vi "CoerceToRange.vi"(10 "Range":T1, 11 "input":dbl) -> (3 "coerced":dbl)   [LabVIEW 2017]
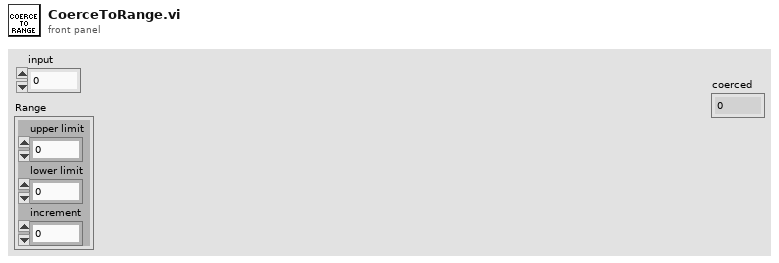
[diagram p1: front panel]
types:
  T1 = cluster{"upper limit":dbl, "lower limit":dbl, "increment":dbl}
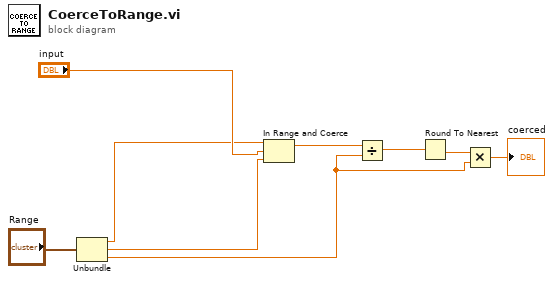
[diagram p0: block diagram]
diagram:
  n1 = Unbundle("Range") -> ("upper limit"=w3:dbl, "lower limit"=w2:dbl, "increment"=w1:dbl)
  n2 = In Range and Coerce(upper limit=w3, x="input", lower limit=w2) -> (coerced(x)=w8:dbl)  [unwired: 1 out]
  n3 = Divide(x=w8, y=w1) -> (x/y=w7:dbl)
  n4 = Round To Nearest(number=w7) -> (nearest integer value=w6:dbl)
  n5 = Multiply(x=w6, y=w1) -> (x*y=→"coerced":dbl)
